vi "Save-sequences-with-dialog.vi"(8 "error in (no error)":errorcluster, 11 "Object ref in":T1) -> (0 "error out":errorcluster, 3 "Object ref out":T1)   [LabVIEW 2013, in "PowderDeposition.lvlib" / "PD-Main.lvclass"]
uses:
  PD-Main.lvclass
  Object-reference.ctl
  PD-Main.lvclass/PD-Main.ctl
  Assembly/Motor-assembly.lvclass
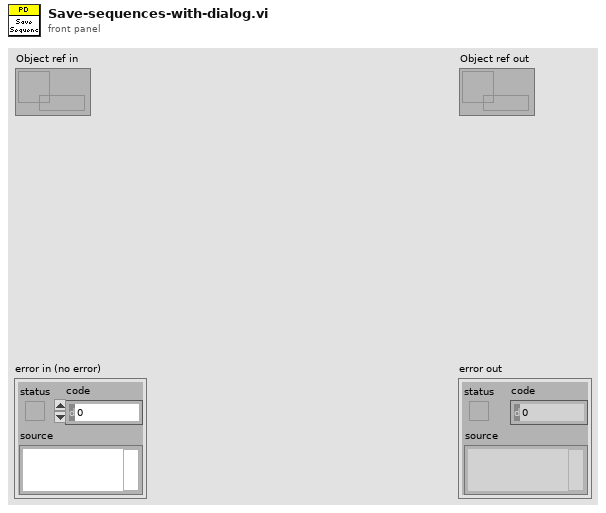
[diagram p1: front panel]
types:
  T1 = typedef "PowderDeposition.lvlib/PD-Main.lvclass/Object-reference.ctl" = refnum<data-value>
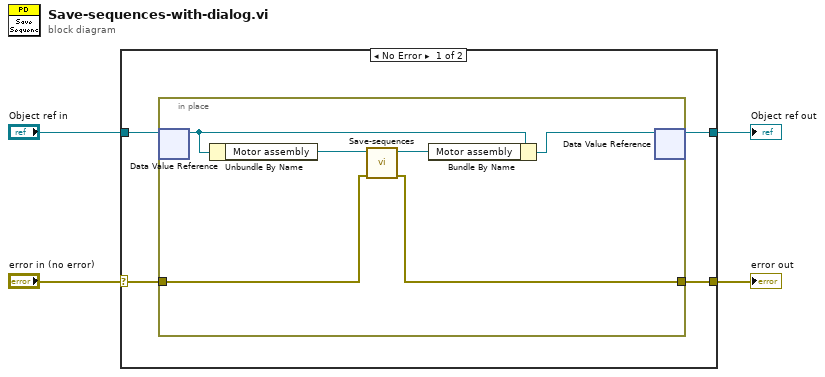
[diagram p0: block diagram]
diagram:
  n1 = case shown="No Error" "error in (no error)" {
    selector: "error in (no error)" -> [w7 w16]
    tunnel: [w6 w16] -> w3
    tunnel: [w5 w15] -> w1
    tunnel: "Object ref in" -> [w8 w15]
    frame No Error {
      n2 = in-place {
        in-place-border: w7 -> [w14]
        in-place-border: [w9] -> w6
        n3 = in-place-dvr #1(w8) -> (w12:refnum<class "PD-Main.lvclass">)  [unwired: 1 out]
        n4 = Unbundle By Name(w12) -> ("Motor assembly"=w13:refnum<class "Motor-assembly.lvclass">)
        n5 = call "Save-sequences.vi"("error in (no error)"=w14, "Available motors in"=w13) -> ("error out"=w9:errorcluster, "Available motors out"=w10:refnum<class "Motor-assembly.lvclass">)  [unwired: 8 in]
        n6 = Bundle By Name(cluster=w12, "Motor assembly"=w10) -> (w11:refnum<class "PD-Main.lvclass">)
        n7 = in-place-dvr #1(w11) -> (w5:T1)  [unwired: 1 out]
      }
    }
    frame Error {
    }
  }
  "error out" <- w3
  "Object ref out" <- w1
